vi "NewChicagoPizzaStore.vi"(8 "error in (no error)":errorcluster) -> (0 "error out":errorcluster, 3 "ChicagoPizzaStore":refnum<class "ChicagoPizzaStore.lvclass">)   [LabVIEW 2020, in "FactoryMethod.lvlib" / "PizzaFactoryMethod.lvlib" / "ChicagoPizzaStore.lvclass"]
uses:
  ChicagoPizzaStore.lvclass
  ChicagoPizzaStore.lvclass/ChicagoPizzaStore.ctl
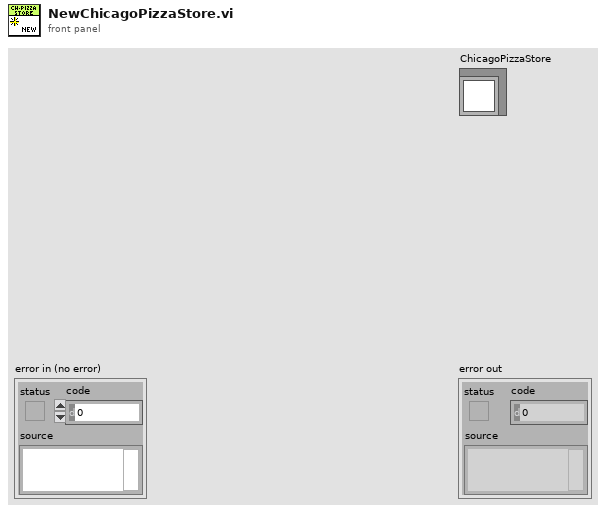
[diagram p1: front panel]
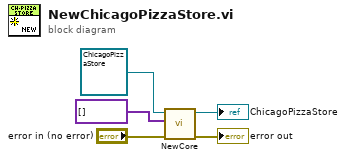
[diagram p0: block diagram]
diagram:
  n1 = call-dynamic "NewCore.vi"("error in (no error)"="error in (no error)", "ParamsArray"=variant[] [], "ChicagoPizzaStore"=refnum<class "ChicagoPizzaStore.lvclass"> refnum ("NYPizzaStore")) -> ("error out"=→"error out":errorcluster, "ChicagoPizzaStore"=→"ChicagoPizzaStore":refnum<class "ChicagoPizzaStore.lvclass">)  [unwired: 7 in]
